vi "simulaVolt.vi"(8 "error in (no error)":errorcluster, 10 "volt in":dbl=0.75 format="%#_13g") -> (0 "error out":errorcluster, 2 "volt out":dbl, 3 "Keithley2002 out":refnum<class "Keithley2002.lvclass">)   [LabVIEW 2019, in "Keithley2002.lvclass"]
uses:
  Keithley2002.lvclass
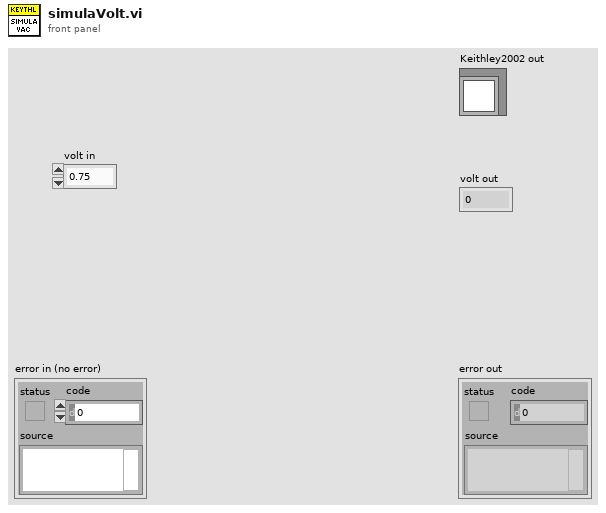
[diagram p1: front panel]
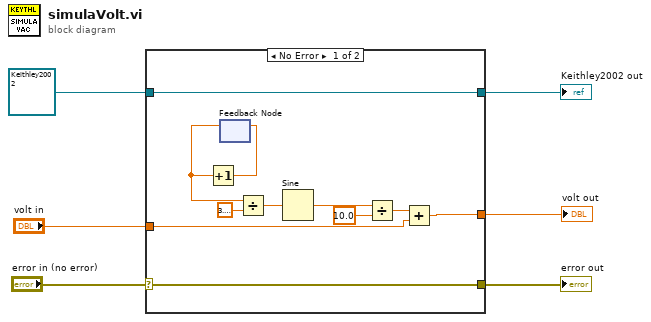
[diagram p0: block diagram]
diagram:
  n1 = case shown="No Error" "error in (no error)" {
    selector: "error in (no error)" -> [w16 w19]
    tunnel: [w16 w19] -> w5
    tunnel: [w17 w18] -> w3
    tunnel: refnum<class "Keithley2002.lvclass"> refnum ("Keithley2002 in") -> [w17 w18]
    tunnel: "volt in" -> [w10 _]
    tunnel: [w9 _] -> w1
    frame No Error {
      n2 = feedback #1() -> (w11:dbl)  [unwired: 1 in]
      n3 = Increment(x=w11) -> (x+1=w15:dbl)
      n4 = feedback-in #1(w15) -> ()
      n5 = Divide(x=w11, y=3.141592653589793) -> (x/y=w14:dbl)
      n6 = Sine(x=w14) -> (sin(x)=w12:dbl)
      n7 = Divide(x=w12, y=10.0) -> (x/y=w8:dbl)
      n8 = Add(x=w8, y=w10) -> (x+y=w9:dbl)
    }
    frame Error {
    }
  }
  "error out" <- w5
  "Keithley2002 out" <- w3
  "volt out" <- w1
